vi "Write RT FIFO.vi"   [LabVIEW 2017, in "Data Sharing Framework Engine.lvlib" / "Engine Interface.lvclass"]
uses:
  Engine Interface.lvclass
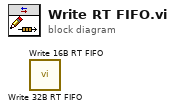
[diagram p0: block diagram]
diagram:
  n1 = call "Write 32B RT FIFO.vi"() -> ()  [unwired: 9 in, 3 out]
  n2 = call "Write 16B RT FIFO.vi"() -> ()  [unwired: 9 in, 3 out]
